vi "UE + DVR storage.vi"() -> ()   [LabVIEW 2017]
doc: "Centralized storage for User events and DVRs used in application"
uses:
  Error/Controls/Error Event.ctl
  Error/Controls/Error Type.ctl
  Configuration/Controls/Config DB Command.ctl
  Configuration/Controls/Config DB Record.ctl
  Controller/Controls/Elevator Location.ctl
  Controller/Controls/Elevator Direction Event.ctl
  Controller/Controls/Elevator Direction.ctl
panel:
  in  "Open/Close Door":refnum<user-event>
  in  "Go to Floor":refnum<user-event>
  in  "Emergency":refnum<user-event>
  in  "DB Record DVR":refnum<data-value>
  in  "DB Command":refnum<user-event>
  in  "Error":refnum<user-event>
  in  "Stop DVR":refnum<data-value>
  in  "Stop":refnum<user-event>
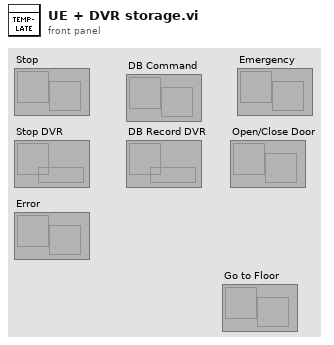
[diagram p1: front panel]
types:
  T1 = typedef "Elevator Direction Event.ctl" = cluster{"Direction":T2, "Departure":T3}
  T2 = typedef "Elevator Direction.ctl" = enum16{"Move Up", "Move Down"}
  T3 = typedef "Elevator Location.ctl" = enum16{"1st Floor", "2nd Floor", "3rd Floor", "4th Floor"}
  T4 = typedef "Config DB Record.ctl" = cluster{"Door Open":dbl, "Door Close":dbl, "Travel Time":dbl, "Inactivity Time":dbl}
  T5 = typedef "Config DB Command.ctl" = enum16{"Read", "Update"}
  T6 = typedef "Error Event.ctl" = cluster{"Error Type":T7, "Description":string, "Date Time":string, "Source":variant}
  T7 = typedef "Error Type.ctl" = enum16{"Console Error", "Sensor Interface IO Error", "Process Step Error"}
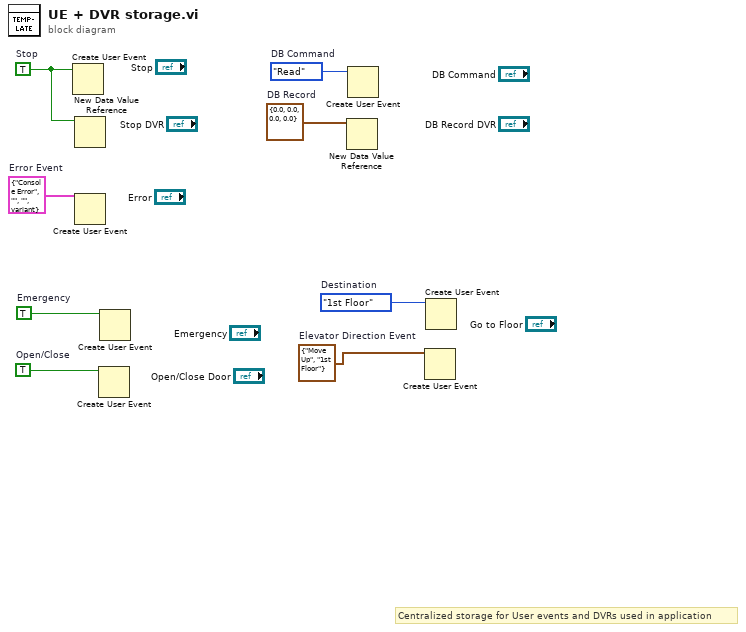
[diagram p0: block diagram]
diagram:
  w1 = T1 {"Direction"=enum."Move Up", "Departure"=enum."1st Floor"}  # Elevator Direction Event
  w2 = Elevator_Location."1st Floor"  # Destination
  w3 = TRUE  # Open/Close
  w4 = TRUE  # Emergency
  w5 = T4 {"Door Open"=0.0, "Door Close"=0.0, "Travel Time"=0.0, "Inactivity Time"=0.0}  # DB Record
  w6 = Config_DB_Command."Read"  # DB Command
  w7 = T6 {"Error Type"=enum."Console Error", "Description"="", "Date Time"="", "Source"=variant}  # Error Event
  w8 = TRUE  # Stop
  # "Centralized storage for User events and DVRs used in application"
  n1 = Create User Event(user event datatype=w8) -> ()  [unwired: 1 in, 2 out]
  n2 = New Data Value Reference(data value=w8) -> ()  [unwired: 1 in, 2 out]
  n3 = Create User Event(user event datatype=w7) -> ()  [unwired: 1 in, 2 out]
  n4 = Create User Event(user event datatype=w3) -> ()  [unwired: 1 in, 2 out]
  n5 = Create User Event(user event datatype=w4) -> ()  [unwired: 1 in, 2 out]
  n6 = New Data Value Reference(data value=w5) -> ()  [unwired: 1 in, 2 out]
  n7 = Create User Event(user event datatype=w6) -> ()  [unwired: 1 in, 2 out]
  n8 = Create User Event(user event datatype=w1) -> ()  [unwired: 1 in, 2 out]
  n9 = Create User Event(user event datatype=w2) -> ()  [unwired: 1 in, 2 out]
